vi "(SubVI)Scope_Sensor Activation.vi"(8 "error in (no error)":errorcluster caption="에러 입력(에러 없음)") -> (0 "error out":errorcluster caption="에러 출력", 3 "Valid":bool[](array[boolean]))   [LabVIEW 2020]
uses:
  Serial/Controls/(Ctrl)Serial_Write Read Option.ctl
  Serial/Controls/(Ctrl)Serial_FGV Function.ctl
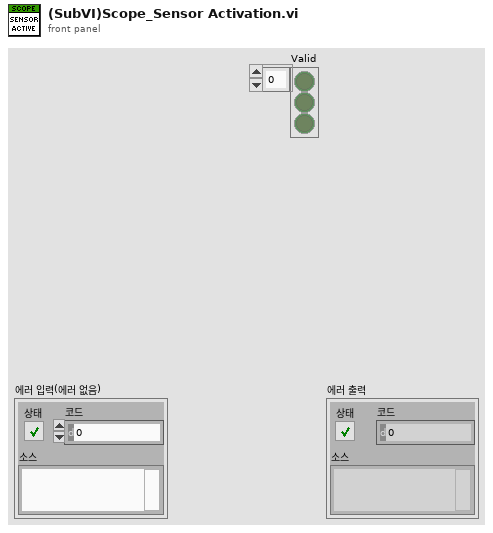
[diagram p1: front panel]
types:
  T1 = typedef "(Ctrl)Serial_Write Read Option.ctl" = cluster{"Echo Request":bool, "Header Verification":bool, "Checksum Verification":bool, "User Code Verifiaction":bool}
  T2 = typedef "(Ctrl)Serial_FGV Function.ctl" = enum16{"Initialize", "Read", "Read All", "Write", "Flush Buffer", "Get Ref.", "Close"}
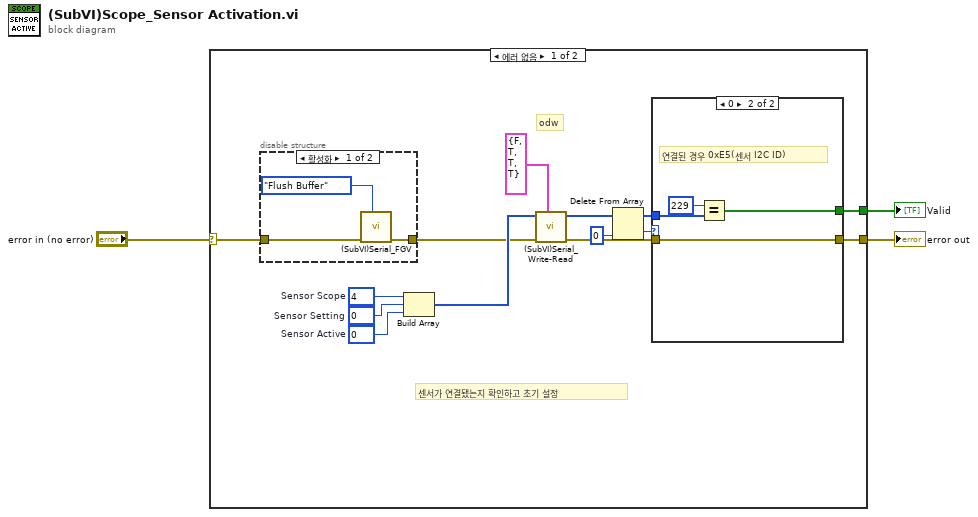
[diagram p0: block diagram]
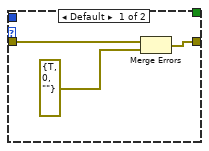
[diagram p3: hidden frame]
diagram:
  n1 = case shown="에러 없음" "error in (no error)" {
    selector: "error in (no error)" -> [w13 w29]
    tunnel: [w14 w29] -> w3
    tunnel: [w5 _] -> w1
    frame No Error {
      w16 = u8 0  # Sensor Setting
      w15 = u8 0  # Sensor Active
      w17 = u8 4  # Sensor Scope
      # "odw"
      # "센서가 연결됐는지 확인하고 초기 설정"
      n2 = disable-structure shown="활성화" {
        disable-tunnel: w13 -> [w20 w21]
        disable-tunnel: [w19 w21] -> w4
        frame Enabled {
          n3 = call "(SubVI)Serial_FGV.vi"("Function"=(Ctrl)Serial_FGV_Function."Flush Buffer", "error in (no error)"=w20) -> ("error out"=w19:errorcluster)  [unwired: 7 in, 2 out]
        }
        frame Disabled {
        }
      }
      n4 = Build Array(w17, w16, w15) -> (w9:u8[])
      n5 = call "(SubVI)Serial_Write-Read.vi"("Option"=T1 {"Echo Request"=FALSE, "Header Verification"=TRUE, "Checksum Verification"=TRUE, "User Code Verifiaction"=TRUE}, "error in (no error)"=w4, "Data to Write"=w9) -> ("error out"=w10:errorcluster, "Read Data"=w11:u8[])  [unwired: 6 in, 1 out]
      n6 = Delete From Array(array=w11, index=0 ("인덱스")) -> (deleted portion=w8:u8, array with subset deleted=w6:u8[])  [unwired: 1 in]
      n7 = case shown="0" w8 {
        tunnel: w10 -> [w24 w28]
        tunnel: [w23 w28] -> w14
        tunnel: w6 -> [_ w27]
        tunnel: [_ w25] -> w5
        frame Default {
          n8 = Merge Errors(w24, errorcluster {"status"=TRUE, "code"=0, "source"=""} ("에러 입력")) -> (w23:errorcluster)
        }
        frame 0 {
          # "연결된 경우 0xE5(센서 I2C ID)"
          n9 = Equal?(x=u8 229 ("숫자형"), y=w27) -> (x = y?=w25:bool[])
        }
      }
    }
    frame Error {
    }
  }
  "error out" <- w3
  "Valid" <- w1
